vi "setCenterWavelength.vi"(6 "Delay between send and receive [ms]":i32=100, 8 "error in (no error)":errorcluster, 9 "monoIndex":i32=1, 10 "wavelength":dbl, 11 "CCD in":refnum<class "CCD.lvclass">) -> (0 "error out":errorcluster, 1 "ID":i32, 2 "results-JSON string":string, 3 "CCD out":refnum<class "CCD.lvclass">)   [LabVIEW 2023, in "horiba.lvlib" / "CCD.lvclass"]
doc: "This command sets the center wavelength value and other parameters to be used in the pixel to wavelength conversion.\n\nNote: This command should be called before ccd_setXAxisConversionType and ccd_setAcquisitionStart and is only useful uf the xAxisConversion type is set to Fitparams."
uses:
  CCD.lvclass
  20f7d3bd-08ac-4524-9bed-df36c1da25a0.vi
  a8db981f-de0e-4bb5-ae19-63df6e2f9c8d.vi
  fbfd7e04-0e37-456c-889d-0219d7529662.vi
  <vilib>/JDP Science/JSONtext/Variant to JSON Text.vi
  <vilib>/JDP Science/JSONtext/Set Item.vi
  <vilib>/JDP Science/JSONtext/LVClass Serializer/JSONtext LVClass Serializer.lvclass
  GenericDevice/GenericDevice.lvclass
panel:
  # "Connector Pane"
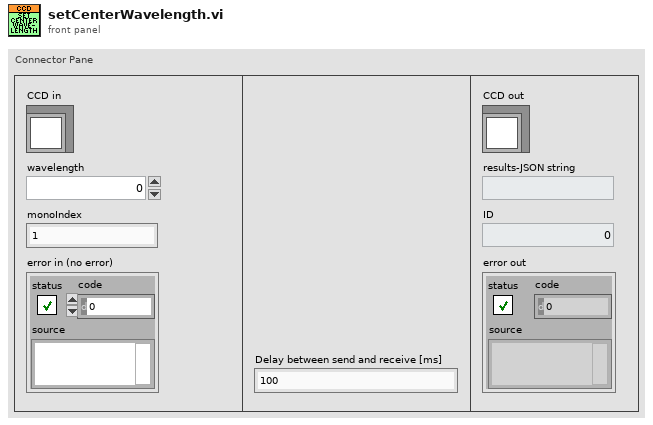
[diagram p1: front panel]
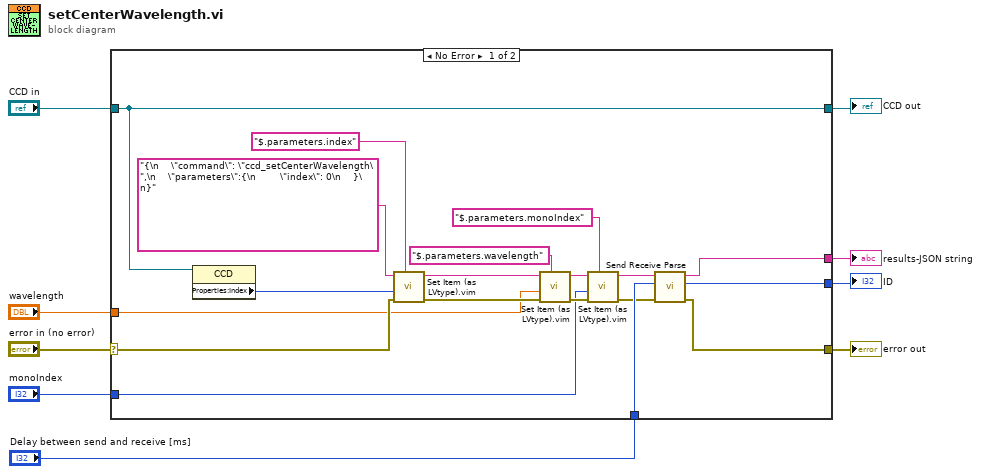
[diagram p0: block diagram]
diagram:
  n1 = case shown="No Error" "error in (no error)" {
    selector: "error in (no error)" -> [w24 w30]
    tunnel: [w18 w30] -> w8
    tunnel: [w26 w29] -> w6
    tunnel: "CCD in" -> [w26 w29]
    tunnel: "wavelength" -> [w16 _]
    tunnel: [w20 _] -> w5
    tunnel: [w19 _] -> w4
    tunnel: "Delay between send and receive [ms]" -> [w17 _]
    tunnel: "monoIndex" -> [w10 _]
    frame No Error {
      n2 = property class="CCD"(reference=w26) -> ("Properties:Index"=w25:i32)  [unwired: 1 in, 2 out]
      n3 = call "Set Item (as LVtype).vim"("$Path or Item Name"="$.parameters.index", "error in (no error)"=w24, "Anything"=w25, "JSON"="{\n    \"command\": \"ccd_setCenterWavelength\",\n    \"parameters\":{\n        \"index\": 0\n    }\n}") -> ("error out"=w22:errorcluster, "<JSON>"=w23:string)  [unwired: 4 in, 1 out]
      n4 = call "Set Item (as LVtype).vim"("$Path or Item Name"="$.parameters.wavelength", "error in (no error)"=w22, "Anything"=w16, "JSON"=w23) -> ("error out"=w14:errorcluster, "<JSON>"=w15:string)  [unwired: 4 in, 1 out]
      n5 = call "Set Item (as LVtype).vim"("$Path or Item Name"="$.parameters.monoIndex", "error in (no error)"=w14, "Anything"=w10, "JSON"=w15) -> ("error out"=w12:errorcluster, "<JSON>"=w13:string)  [unwired: 4 in, 1 out]
      n6 = call "Send Receive Parse.vi"("error in"=w12, "Delay between send and receive [ms]"=w17, "<JSON>"=w13) -> ("error out"=w18:errorcluster, "ID"=w19:i32, "results-JSON string"=w20:string)  [unwired: 6 in]
    }
    frame Error {
    }
  }
  "error out" <- w8
  "CCD out" <- w6
  "results-JSON string" <- w5
  "ID" <- w4
